vi "Configure Smoothing Parameter.vi"(4 "Smooth Aperture (25.0)":dbl=25.0 format="%.2p", 5 "Mode (0: Smooth Points)":u16(ring) items=["Smooth Points", "Smooth Aperture"], 6 "Smooth Points (1)":i32=1, 7 "Smooth State (F: Off)":bool, 8 "Error In (no error)":errorcluster, 9 "Measurement Name (MY_MEAS)":string="MY_MEAS", 10 "Channel (1)":i32=1, 11 "VISA Resource Name":refnum<visa-resource-name>) -> (0 "Error Out":errorcluster, 3 "VISA Resource Name Out":refnum<visa-resource-name>)   [LabVIEW 2018, in "Agilent PNA Series.lvlib"]
doc: "This VI sets the smoothing state and number of adjacent data points to average for the selected channel and measurement or the amount of smoothing as a ratio of number of data points in the measurement trace."
uses:
  Agilent PNA Series.lvlib
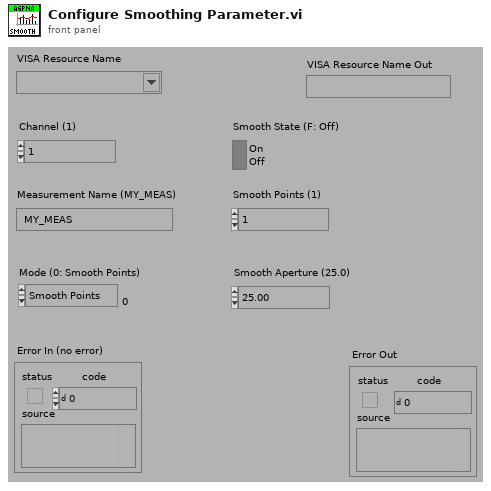
[diagram p1: front panel]
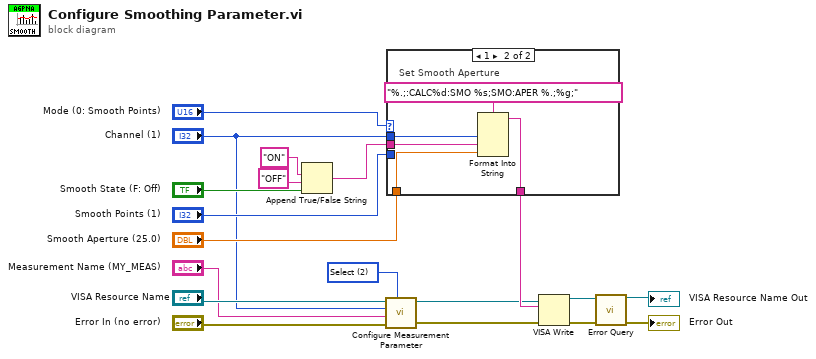
[diagram p0: block diagram]
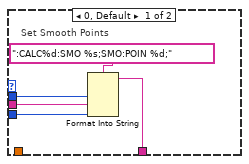
[diagram p2: hidden frame]
diagram:
  w8 = u16 2 items=["Create", "Delete", "Select"] ("Mode (0: Create)")
  n1 = Append True/False String(1:"Smooth State (F: Off)", 2:"OFF" ("f"), 3:"ON") -> (0:w17:string)  [unwired: 1 in]
  n2 = call "Configure Measurement Parameter.vi"("Mode (0: Create)"=w8, "Error In (no error)"="Error In (no error)", "Measurement Name (MY_MEAS)"="Measurement Name (MY_MEAS)", "Channel (1)"="Channel (1)", "VISA Resource Name"="VISA Resource Name") -> ("Error Out"=w12:errorcluster, "VISA Resource Name Out"=w5:refnum<visa-resource-name>)  [unwired: 5 in]
  n3 = case shown="1" "Mode (0: Smooth Points)" {
    tunnel: [w24 w29] -> w6
    tunnel: "Channel (1)" -> [w23 w28]
    tunnel: w17 -> [w21 w26]
    tunnel: "Smooth Points (1)" -> [w20 _]
    tunnel: "Smooth Aperture (25.0)" -> [_ w25]
    frame 0, Default {
      # "Set Smooth Points"
      n4 = Format Into String(format string=":CALC%d:SMO %s;SMO:POIN %d;", w23, w21, w20) -> (resulting string=w24:string)  [unwired: 2 in, 1 out]
    }
    frame 1 {
      # "Set Smooth Aperture"
      n5 = Format Into String(format string="%.;:CALC%d:SMO %s;SMO:APER %.;%g;", w28, w26, w25) -> (resulting string=w29:string)  [unwired: 2 in, 1 out]
    }
  }
  n6 = VISA Write(VISA resource name=w5, write buffer=w6, error in (no error)=w12) -> (VISA resource name out=w4:refnum<visa-resource-name>, error out=w3:errorcluster)  [unwired: 1 out]
  n7 = call "Error Query.vi"("VISA Resource Name"=w4, "error in (no error)"=w3) -> ("VISA Resource Name Out"=→"VISA Resource Name Out":refnum<visa-resource-name>, "error out"=→"Error Out":errorcluster)  [unwired: 10 in, 2 out]
